vi "Perform Audio Measurements.vi"(0 "Measurement Configuration":T1={"Band start"=20.0, "Band stop"=20000.0, "Weighting filter"=0, "Full scale range"=3.16, "Analog source resource name"="", "Frequency"=1000.0, "Amplitude"=1.0, "Protocol capture resource name"="PXI1Slot7\\I2Si 0", "Protocol capture channel"="", "Clock rate"=12288000, "Number of words"=19200, "Sensitivity"=0.34762, "JSONFile"=""}, 2 "PCM waveforms":waveform(dbl)[](array[waveform]), 3 "error in (no error)":errorcluster) -> (7 "Measurement Results":T2, 10 "error out":errorcluster)   [LabVIEW 2021, in "audio_acMeasurement.lvlib"]
uses:
  audio_acMeasurement.lvlib
  Measurement Results.ctl
  Measurement Configuration.ctl
  <vilib>/addons/_NISVFA/_Shared subVIs/Controls/svc_Window.ctl
  <vilib>/addons/_NISVFA/_Shared subVIs/Common/SVL Set dB Reference (N Ch - 1 Ref).vi
  <vilib>/addons/Sound and Vibration/svt_Level/SVL AC & DC Level (Time) (N Ch).vi
  <vilib>/addons/Sound and Vibration/svt_Single Tone Measurements/SVT Spurious Free Dynamic Range (Frequency) (1 Ch).vi
  <vilib>/addons/_NISVFA/_Spectrum Processing/SVFA Unit Conversion (Complex) (1 Ch).vi
  <vilib>/addons/_NISVFA/_Shared subVIs/Common/SVL Set dB Reference (1 Ch).vi
  <vilib>/addons/Sound and Vibration/svt_Level/SVL AC & DC Level (Time) (1 Ch).vi
  <vilib>/addons/_NISVFA/_Spectrum Processing/SVFA Get Spectrum Subset.vi
  <vilib>/addons/_NISVFA/_Spectrum Processing/SVFA Get Spectrum Subset (Complex) (1 Ch).vi
  <vilib>/addons/_NISVFA/_Shared subVIs/Common/svc_Window Parameters.vi
  <vilib>/addons/_NISVFA/_Shared subVIs/Common/svc_Extract Single Tone Information (complex).vi
  <vilib>/addons/_NISVFA/_Shared subVIs/Common/svc_Check Frequency Range in Spectrum.vi
  <vilib>/addons/_NISVFA/_Spectrum Processing/SVFA Spectrum Peak Search.vi
  <vilib>/addons/_NISVFA/_Spectrum Processing/SVFA Spectrum Peak Search (1 Ch).vi
  <vilib>/addons/_NISVFA/_Shared subVIs/Common/svc_Spectrum Units.vi
  <vilib>/addons/_NISVFA/_Shared subVIs/Common/svc_Log View for Spectrum (1Ch).vi
  <vilib>/addons/_NISVFA/_Spectrum Processing/SVFA Unit Conversion (1 Ch).vi
  <vilib>/addons/_NISVFA/_Shared subVIs/Common/svc_Complex Datatype Defaults.vi
  <vilib>/addons/_NISVFA/_Shared subVIs/Common/svc_Build Unit Label for Frequency Range.vi
  <vilib>/addons/_NISVFA/_Shared subVIs/Common/SVL Set dB Reference (variant).vi
  <vilib>/addons/_NISVFA/_Shared subVIs/Common/svc_Get SV Channel Info.vi
  <vilib>/Analysis/baseanly.llb/Mean.vi
  <vilib>/Analysis/baseanly.llb/Mean (DBL).vi
  <vilib>/addons/_NISVFA/_Shared subVIs/Windowing/svfa_Scaled Time Domain Window (Array).vi
  <vilib>/addons/_NISVFA/_Spectrum Processing/SVFA Get Tone Amplitude and Phase (1 Ch).vi
  <vilib>/addons/_NISVFA/_Spectrum Processing/subVIs/svfa_Compute Complex Spectrum for Export.vi
  <vilib>/addons/_NISVFA/_Shared subVIs/Common/svc_Check Frequency Range in Bandwidth.vi
  <vilib>/addons/_NISVFA/_Shared subVIs/Common/svc_Convert Start and Stop to Start Index and Length.vi
  <vilib>/addons/_NISVFA/_Spectrum Processing/subVIs/svfa_Spectrum Peak Search.vi
  <vilib>/addons/_NISVFA/_Shared subVIs/Common/svc_Format Value (DBL).vi
  <vilib>/addons/_NISVFA/_Shared subVIs/Common/svc_Get Weighting Enum and Labels.vi
  <vilib>/addons/_NISVFA/_Shared subVIs/Common/svc_Engineering Units to Unit Label.vi
  <vilib>/addons/_NISVFA/_Shared subVIs/Common/svc_Surround NonAlpha String with Parentheses.vi
  <vilib>/dlg_ctls.llb/Space Constant.vi
  <vilib>/addons/_NISVFA/_Shared subVIs/Common/svc_Unwrap Phase.vi
  <vilib>/addons/_NISVFA/_Shared subVIs/Common/svc_Convert Spectrum Array to dB.vi
  <vilib>/addons/_NISVFA/_Spectrum Processing/subVIs/svfa_Conversion Utility (spectrum info).vi
  <vilib>/addons/_NISVFA/_Shared subVIs/Common/svc_Unit Label to Engineering Units.vi
  <vilib>/addons/_NISVFA/_Spectrum Processing/subVIs/svfa_Spectrum Info Window to windowTd Type Def.vi
  <vilib>/Analysis/4window.llb/Force Window.vi
  <vilib>/Analysis/4window.llb/Force Window (DBL).vi
  <vilib>/Analysis/4window.llb/Exponential Window.vi
  <vilib>/Analysis/4window.llb/Exponential Window (DBL).vi
  <vilib>/addons/_NISVFA/_Spectrum Processing/subVIs/svfa_Window Frequency Response.vi
  <vilib>/addons/_NISVFA/_Spectrum Processing/subVIs/svfa_Window Frequency Response (double array).vi
  <vilib>/Analysis/baseanly.llb/Dot Product.vi
  <vilib>/Analysis/baseanly.llb/Complex Dot Product.vi
  <vilib>/addons/_NISVFA/_Spectrum Processing/subVIs/svfa_Peak Rough Search Indices.vi
  <vilib>/addons/_NISVFA/_Shared subVIs/Common/svc_Unit Label Lexical Class.vi
  <vilib>/addons/_NISVFA/_Spectrum Processing/subVIs/svfa_Peak to RMS to Peak2Peak.vi
  <vilib>/addons/_NISVFA/_Spectrum Processing/subVIs/svfa_Mag to Mag2.vi
  <vilib>/addons/_NISVFA/_Spectrum Processing/subVIs/svfa_Linear to dB.vi
  <vilib>/addons/_NISVFA/_Spectrum Processing/subVIs/svfa_dBrefA to dBrefB.vi
  <vilib>/addons/_NISVFA/_Spectrum Processing/subVIs/svfa_Spectrum to Spectral Density.vi
  <vilib>/addons/_NISVFA/_Spectrum Processing/subVIs/svfa_Rect Window Frequency Response.vi
  <vilib>/addons/_NISVFA/_Spectrum Processing/subVIs/svfa_Cosine Window Coefficients.vi
  <vilib>/measure/matone.llb/Extract Single Tone Information N Chan.vi
  <vilib>/addons/Sound and Vibration/svt_Weighting/SVT Weighting Filter (N Ch).vi
  <vilib>/addons/_NISVFA/_Shared subVIs/Common/svc_Caller VI Returned in Error Source.vi
  <vilib>/addons/_NISVFA/_Shared subVIs/Common/svc_Get Window Info.vi
  <vilib>/Analysis/0measdsp.llb/Scaled Time Domain Window.vi
  <vilib>/Analysis/0measdsp.llb/Scaled Time Domain Window (DBL).vi
  <vilib>/Utility/error.llb/Error Cluster From Error Code.vi
  <vilib>/Analysis/baseanly.llb/Std Deviation and Variance.vi
  <vilib>/addons/Sound and Vibration/svt_Single Tone Measurements/SVT Gain (Time) (1 Ch).vi
  <vilib>/addons/Sound and Vibration/svt_Distortion/SVT SNR without Harmonics (Frequency) (1 Ch).vi
  <vilib>/addons/Sound and Vibration/svt_Single Tone Measurements/SVT Dynamic Range (Frequency) (1 Ch).vi
  <vilib>/addons/Sound and Vibration/svt_Distortion/subVIs/sv_Check Data Valid (Audio) (1 Ch).vi
  <vilib>/addons/_NISVFA/_Shared subVIs/Common/svc_Convert Frequency to Frequency String.vi
  <vilib>/Analysis/4window.llb/window parameters.vi
  <vilib>/Analysis/4window.llb/Window Properties.vi
  <vilib>/Analysis/4window.llb/Window Properties by Name.vi
  <vilib>/addons/_NISVFA/_Spectrum Processing/subVIs/svfa_Spectrum Peak Tone Search and Estimation (complex).vi
  <vilib>/measure/masignal.llb/Tones and Noise Waveform.vi
  <vilib>/addons/_NISVFA/_Shared subVIs/Common/svc_FFT with Window.vi
  <vilib>/Analysis/1siggen.llb/Square Wave.vi
  <vilib>/addons/_NISVFA/_Spectrum Processing/subVIs/svfa_Three Finger Peak Search.vi
  <vilib>/addons/Sound and Vibration/svt_Distortion/subVIs/sv_Peak View Amplitude (1 Ch).vi
  <vilib>/addons/Sound and Vibration/svt_Single Tone Measurements/SoundVib_SingleTone.lvlib
  <vilib>/addons/Sound and Vibration/svt_Distortion/SoundVib_Distortion.lvlib
  <vilib>/addons/Sound and Vibration/svt_Weighting/SoundVib_ABCWeighting.lvlib
  <vilib>/measure/NI_MAPro.lvlib
panel:
  out "detected amplitudes":dbl[](array[numeric]) format="%.2p"
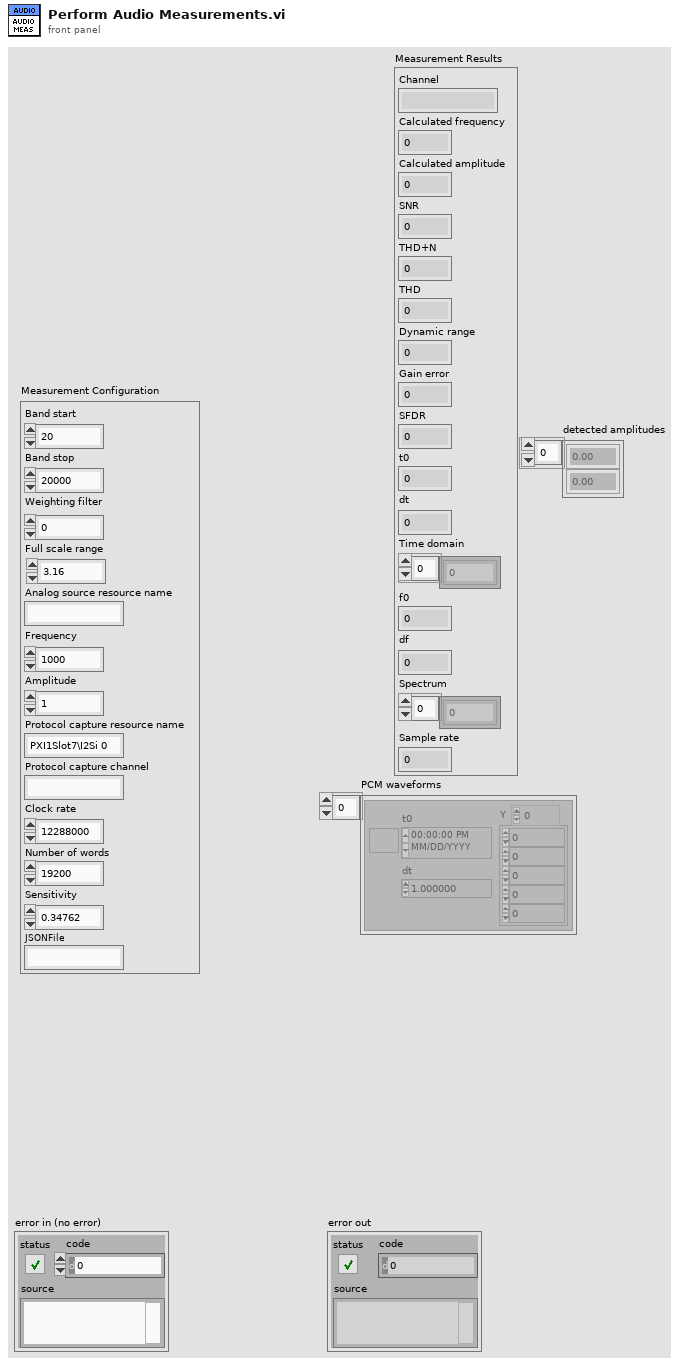
[diagram p1: front panel]
types:
  T1 = typedef "audio_acMeasurement.lvlib/Measurement Configuration.ctl" = cluster{"Band start":dbl, "Band stop":dbl, "Weighting filter":u16, "Full scale range":dbl, "Analog source resource name":string, "Frequency":dbl, "Amplitude":dbl, "Protocol capture resource name":string, "Protocol capture channel":string, "Clock rate":u32, "Number of words":u32, "Sensitivity":dbl, "JSONFile":string}
  T2 = typedef "audio_acMeasurement.lvlib/Measurement Results.ctl" = cluster{"Channel":string, "Calculated frequency":dbl, "Calculated amplitude":dbl, "SNR":dbl, "THD+N":dbl, "THD":dbl, "Dynamic range":dbl, "Gain error":dbl, "SFDR":dbl, "t0":dbl, "dt":dbl, "Time domain":dbl[], "f0":dbl, "df":dbl, "Spectrum":dbl[], "Sample rate":u32}
  T3 = enum16{"no change", "spectrum", "spectral density"}
  T4 = cluster{"linear/dB":enum16{"no change", "linear", "dB"}, "dB reference (0: no change)":dbl, "power/magnitude":enum16{"no change", "power", "magnitude"}, "view":enum16{"no change", "rms", "peak", "peak-peak"}}
  T5 = cluster{"start frequency":dbl, "stop frequency":dbl}
  T6 = cluster{"gain units":enum16{"dB", "linear ratio"}, "detected fundamental amplitude units":enum16{"EU rms", "EU peak", "EU peak-peak"}}
  T7 = typedef "svc_Window.ctl" = u32
  T8 = cluster{"SNR units":enum16{"dB", "linear ratio", "%"}, "detected fundamental amplitude units":enum16{"EU rms", "EU peak", "EU peak-peak"}}
  T9 = typedef "svc_Spectrum Info.ctl" = cluster{"channel name":string, "description":string, "x-axis units":T10, "spectral info":cluster{"spectrum type":T11, "linear/dB":enum16{"linear", "dB"}, "window":u16, "window size":i32, "FFT size":i32}, "engineering units":T12, "custom label":string, "dB reference [EU]":dbl, "peak units":enum16{"rms", "peak", "peak-peak"}, "weighting filter":T13, "spectral density?":bool, "unit label":string, "spectrum skewed?":bool, "complimentary spectrum units":T14}
  T10 = typedef "svc_X-Axis Units.ctl" = u16
  T11 = typedef "svc_Spectrum Type.ctl" = enum16{"FFT Spectrum [complex]", "Amplitude [Magnitude]", "Power [Magnitude^2]", "Cross Spectrum [complex]", "Frequency Response [Complex]"}
  T12 = typedef "svc_Engineering Units Text Ring.ctl" = u16
  T13 = typedef "svc_Weighting Filter Text Ring.ctl" = u16
  T14 = typedef "svc_Complimentary Spectrum Units.ctl" = enum16{"none", "radians", "degrees", "cycles", "imaginary"}
  T15 = cluster{"complex spectrum response":cluster{"f0":dbl, "df":dbl, "complex spectrum":cdb[]}, "spectrum info":T9}
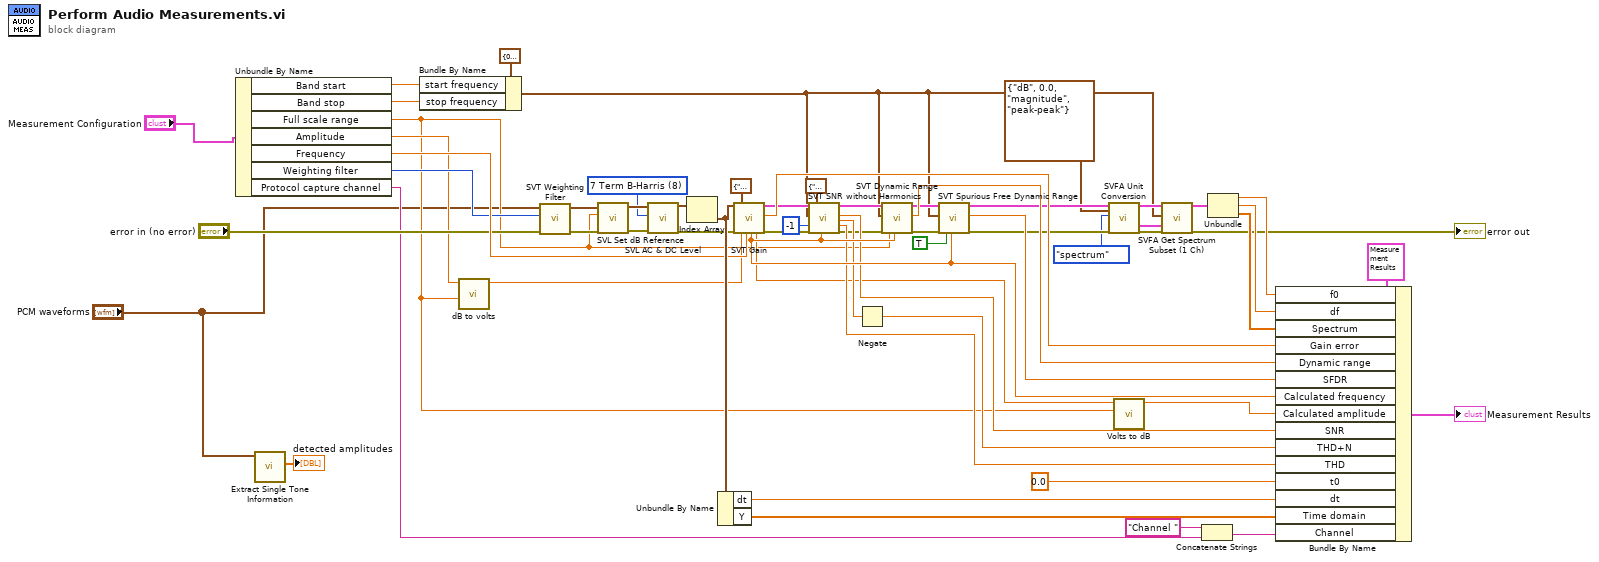
[diagram p0: block diagram]
diagram:
  w29 = T7 8 items=["None"=0, "Hanning"=1, "Hamming"=2, "Blackman-Harris"=3, "Exact Blackman"=4, "Blackman"=5, "Flat Top"=6, "4 Term B-Harris "=7, "7 Term B-Harris"=8, "Low Sidelobe"=9, "Force"=64, "Exponential"=65, "Blackman Nuttall"=11, "Triangle"=30, "Bartlett-Hanning"=31, "Bohman"=32, "Parzen"=33, "Welch"=34, "Kaiser"=60, "Dolph-Chebyshev"=61, "Gaussian"=62] ("window")
  n1 = Unbundle By Name("Measurement Configuration") -> ("Band start"=w46:dbl, "Band stop"=w47:dbl, "Full scale range"=w14:dbl, "Amplitude"=w18:dbl, "Frequency"=w48:dbl, "Weighting filter"=w27:u16, "Protocol capture channel"=w5:string)
  n2 = call-poly <vilib>:"Extract Single Tone Information.vi"("time signals in"="PCM waveforms") -> ("detected amplitudes"=→"detected amplitudes":dbl[])  [unwired: 5 in, 5 out]
  n3 = Bundle By Name(cluster=T5 {"start frequency"=0.0, "stop frequency"=0.0} ("frequency range"), "start frequency"=w46, "stop frequency"=w47) -> (w11:T5)
  n4 = call "dB to volts.vi"("Full scale range"=w14, "Voltage(dB)"=w18) -> ("Voltage(volts)"=w17:dbl)  [unwired: 9 in]
  n5 = call-poly <vilib>:"SVT Weighting Filter.vi"("error in (no error)"="error in (no error)", "weighting"=w27, "scaled signals [EU]"="PCM waveforms") -> ("error out"=w43:errorcluster, "weighted signals [EU]"=w42:waveform(dbl)[])  [unwired: 6 in]
  n6 = call-poly <vilib>:"SVL Set dB Reference.vi"("error in (no error)"=w43, "dB reference [EU]"=w14, "scaled signals in [EU]"=w42) -> ("error out"=w30:errorcluster, "scaled signals out [EU]"=w32:waveform(dbl)[])  [unwired: 7 in]
  n7 = call-poly <vilib>:"SVL AC & DC Level.vi"("scaled signals in [EU]"=w32, "window"=w29, "error in (no error)"=w30) -> ("AC signals [EU]"=w31:waveform(dbl)[], "error out"=w38:errorcluster)  [unwired: 11 in, 4 out]
  n8 = Index Array(array=w31) -> (element=w57:waveform(dbl))  [unwired: 1 in]
  n9 = Unbundle By Name(w57) -> ("dt"=w59:dbl, "Y"=w60:dbl[])
  n10 = call-poly <vilib>:"SVT Gain.vi"("scaled signal [EU]"=w57, "error in (no error)"=w38, "desired units"=T6 {"gain units"=enum."dB", "detected fundamental amplitude units"=enum."EU peak"}, "amplitude [EU peak]"=w17, "expected fundamental frequency [Hz]"=w48) -> ("detected fundamental\nfrequency [Hz]"=w56:dbl, "detected fundamental\namplitude"=w16:dbl, "complex spectrum"=w26:T15, "gain"=w50:dbl, "error out"=w28:errorcluster)  [unwired: 9 in, 1 out]
  n11 = call-poly <vilib>:"SVT SNR without Harmonics.vi"("complex spectrum"=w26, "frequency range"=w11, "maximum harmonic"=-1, "error in (no error)"=w28, "desired units"=T8 {"SNR units"=enum."dB", "detected fundamental amplitude units"=enum."EU rms"}, "expected fundamental frequency [Hz]"=w56) -> ("complex spectrum"=w34:T15, "SNR (without harmonics)"=w53:dbl, "SINAD"=w35:dbl, "THD"=w55:dbl, "error out"=w33:errorcluster)  [unwired: 6 in, 3 out]
  n12 = Negate(x=w35) -> (-x=w54:dbl)
  n13 = call-poly <vilib>:"SVT Dynamic Range.vi"("complex spectrum"=w34, "frequency range"=w11, "error in (no error)"=w33, "full scale amplitude [EU peak]"=w14, "expected fundamental\nfrequency [Hz]"=w56) -> ("dup complex spectrum"=w39:T15, "dynamic range"=w51:dbl, "error out"=w40:errorcluster)  [unwired: 9 in, 3 out]
  n14 = call-poly <vilib>:"SVT Spurious Free Dynamic Range.vi"("complex spectrum"=w39, "frequency range"=w11, "error in (no error)"=w40, "exclude harmonics"=TRUE, "expected fundamental\nfrequency [Hz]"=w56) -> ("complex spectrum"=w24:T15, "spurious free dynamic range"=w52:dbl, "error out"=w25:errorcluster)  [unwired: 7 in, 5 out]
  n15 = call-poly <vilib>:"SVFA Unit Conversion.vi"("complex spectrum"=w24, "desired scaling"=T4 {"linear/dB"=enum."dB", "dB reference (0: no change)"=0.0, "power/magnitude"=enum."magnitude", "view"=enum."peak-peak"}, "spectral density desired"=T3."spectrum", "error in (no error)"=w25) -> ("converted spectrum"=w12:cluster{"x0":dbl, "dx":dbl, "magnitude":dbl[]}, "spectrum info out"=w8:T9, "error out"=w7:errorcluster)  [unwired: 10 in, 3 out]
  n16 = call "Volts to dB.vi"("Full scale range"=w14, "Voltage(V)"=w16) -> ("Voltage(dB)"=w15:dbl)  [unwired: 9 in]
  n17 = call <vilib>:"SVFA Get Spectrum Subset (1 Ch).vi"("spectrum"=w12, "range"=w11, "spectrum info"=w8, "error in (no error)"=w7) -> ("spectrum subset"=w10:cluster{"x0":dbl, "dx":dbl, "magnitude":dbl[]}, "error out"=→"error out":errorcluster)  [unwired: 10 in, 4 out]
  n18 = Concatenate Strings("Channel " ("Channel"), w5) -> (w6:string)
  n19 = Unbundle(w10) -> ("x0"=w21:dbl, "dx"=w20:dbl, "magnitude"=w19:dbl[])
  n20 = Bundle By Name(cluster=T2 {"Channel"="", "Calculated frequency"=0.0, "Calculated amplitude"=0.0, "SNR"=0.0, "THD+N"=0.0, "THD"=0.0, "Dynamic range"=0.0, "Gain error"=0.0, "SFDR"=0.0, "t0"=0.0, "dt"=0.0, "Time domain"=[], "f0"=0.0, "df"=0.0, "Spectrum"=[], "Sample rate"=0} ("Measurement Results"), "f0"=w21, "df"=w20, "Spectrum"=w19, "Gain error"=w50, "Dynamic range"=w51, "SFDR"=w52, "Calculated frequency"=w56, "Calculated amplitude"=w15, "SNR"=w53, "THD+N"=w54, "THD"=w55, "t0"=0.0 ("Wfm t0"), "dt"=w59, "Time domain"=w60, "Channel"=w6) -> (→"Measurement Results":T2)
